vi "Write Nitro.vi"(10 "Nitro":bool, 11 "FPGA API in":refnum<class "FPGA API.lvclass">) -> (3 "FPGA API out":refnum<class "FPGA API.lvclass">)   [LabVIEW 2019, in "FPGA API.lvclass"]
uses:
  FPGA API.lvclass
  FPGA API.lvclass/FPGA API.ctl
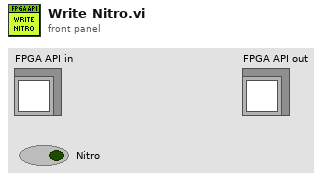
[diagram p1: front panel]
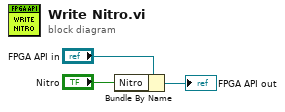
[diagram p0: block diagram]
diagram:
  n1 = Bundle By Name(cluster="FPGA API in", "Nitro"="Nitro") -> (→"FPGA API out":refnum<class "FPGA API.lvclass">)
